vi "Queue_Management_AMC_ALT.vi"(6 "queue error in":errorcluster, 8 "system error in":errorcluster, 9 "Case":string, 10 "Elementos a cola":string[](array[string]), 11 "message queue in":T1) -> (0 "system error out":errorcluster, 2 "elements in queue":cluster{"Estado":string, "Dato":string}[](array[cluster]), 3 "message queue out":T1, 4 "queue error out":errorcluster)   [LabVIEW 2017]
uses:
  <vilib>/NI/AMC/Message Queue.ctl
  <vilib>/NI/AMC/Message.ctl
  <vilib>/NI/Tools/Keyed Array/KeyedArray.ctl
  <vilib>/NI/AMC/Create Single Message.vi
  <vilib>/NI/AMC/Update Message Routing Info.vi
  <vilib>/NI/AMC/Send Message.vi
  <vilib>/NI/AMC/AMC.lvlib
  <vilib>/NI/Tools/Keyed Array/Tools_KeyedArray.lvlib
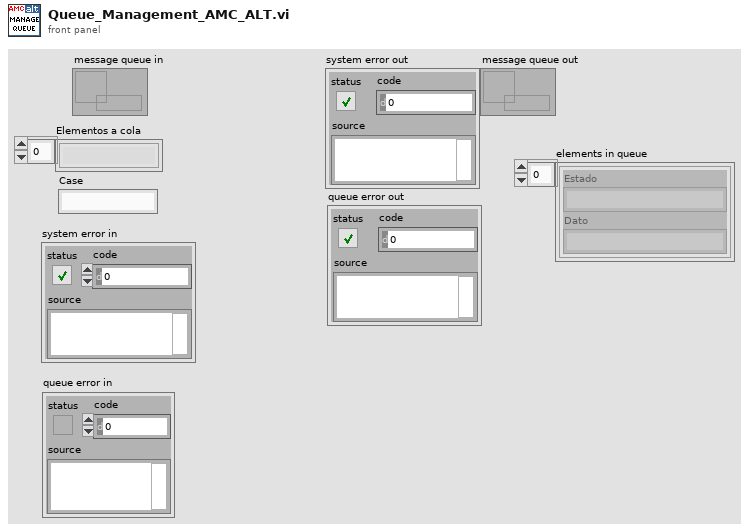
[diagram p1: front panel]
types:
  T1 = typedef "AMC.lvlib/Message Queue.ctl" = refnum<queue>
  T2 = typedef "AMC.lvlib/Message.ctl" = cluster{"name":string, "value":string, "attributes":T3, "receiver host":string, "receiver process":string, "source host":string, "source process":string, "priority message":bool, "acknowledge message":bool}
  T3 = typedef "Tools_KeyedArray.lvlib/KeyedArray.ctl" = cluster{"keys":string[], "values":string[]}
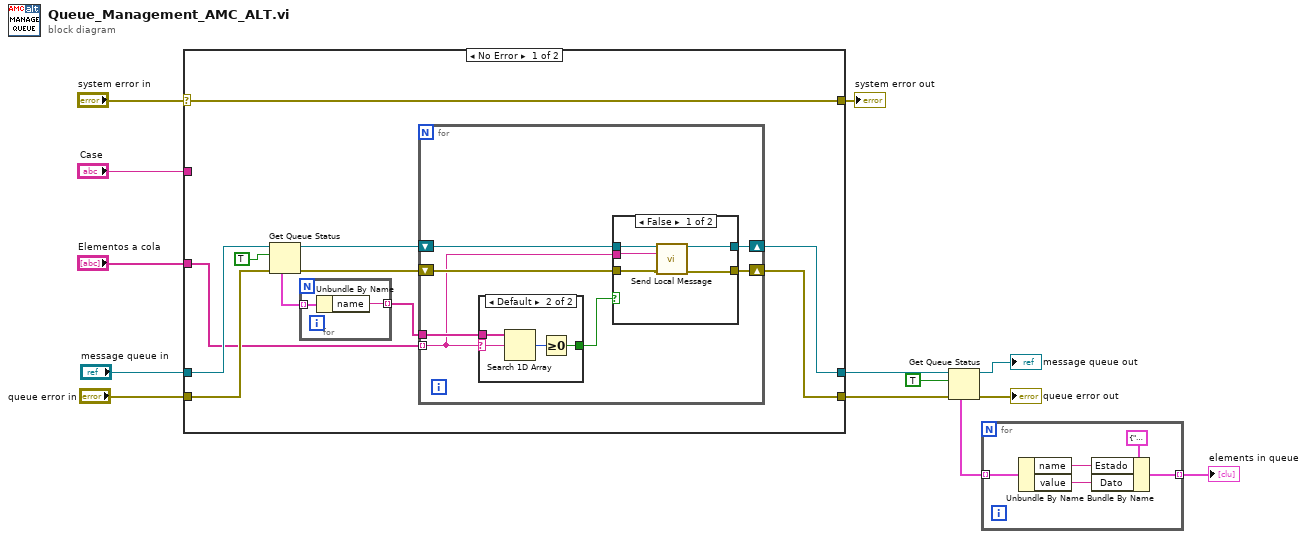
[diagram p0: block diagram]
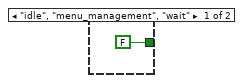
[diagram p2: hidden frame]
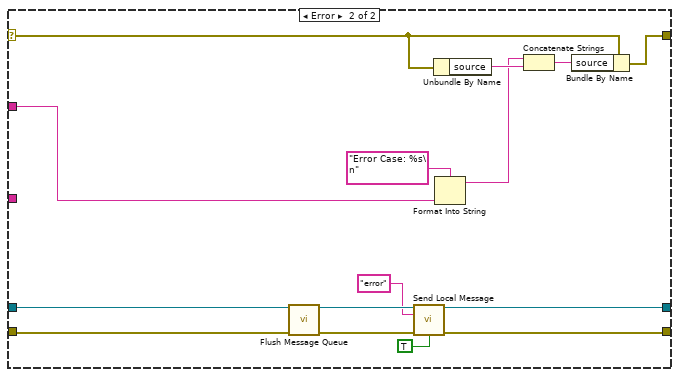
[diagram p4: hidden frame]
diagram:
  n1 = case shown="No Error" "system error in" {
    selector: "system error in" -> [w22 w55]
    tunnel: [w23 w50] -> w4
    tunnel: "Elementos a cola" -> [w16 _]
    tunnel: "message queue in" -> [w18 w52]
    tunnel: [w24 w48] -> w5
    tunnel: "queue error in" -> [w20 w53]
    tunnel: [w22 w56] -> w8
    tunnel: "Case" -> [_ w54]
    frame No Error {
      n2 = Get Queue Status(queue=w18, return elements? (F)=TRUE, error in (no error)=w20) -> (queue out=w17:T1, error out=w19:errorcluster, elements=w15:T2[])  [unwired: 5 out]
      n3 = for {
        tunnel: w15 -> [w26] mode=indexing
        tunnel: [w25] -> w14 mode=indexing
        n4 = Unbundle By Name(w26) -> ("name"=w25:string)
      }
      n5 = for {
        shift-right: [w33] -> w24
        shift-left: w17 -> [w32]
        shift-right: [w30] -> w23
        shift-left: w19 -> [w31]
        tunnel: w14 -> [w28]
        tunnel: w16 -> [w27] mode=indexing
        n6 = case shown="Default" w27 {
          selector: w27 -> [_ w35]
          tunnel: [FALSE w38] -> w29
          tunnel: w28 -> [_ w36]
          frame "idle", "menu_management", "wait" {
          }
          frame Default {
            n7 = Search 1D Array(1D array=w36, element=w35) -> (index of element=w37:i32)  [unwired: 1 in]
            n8 = Greater Or Equal To 0?(x=w37) -> (x >= 0?=w38:bool)
          }
        }
        n9 = case shown="False" w29 {
          tunnel: [w40 w45] -> w33
          tunnel: w32 -> [w43 w45]
          tunnel: w31 -> [w42 w44]
          tunnel: [w39 w44] -> w30
          tunnel: w27 -> [w41 _]
          frame False {
            n10 = call <vilib>:"Send Local Message.vi"("message queue in"=w43, "message name"=w41, "error in"=w42) -> ("message queue out"=w40:T1, "error out"=w39:errorcluster)  [unwired: 10 in, 1 out]
          }
          frame True {
          }
        }
      }
    }
    frame Error {
      n11 = call <vilib>:"Flush Message Queue.vi"("message queue in"=w52, "error in"=w53) -> ("message queue out"=w49:T1, "error out"=w51:errorcluster)  [unwired: 11 in, 1 out]
      n12 = call <vilib>:"Send Local Message.vi"("message queue in"=w49, "message name"="error" ("element"), "error in"=w51, "priority message (F)"=TRUE) -> ("message queue out"=w48:T1, "error out"=w50:errorcluster)  [unwired: 9 in, 1 out]
      n13 = Unbundle By Name(w55) -> ("source"=w59:string)
      n14 = Format Into String(format string="Error Case: %s\n", w54) -> (resulting string=w58:string)  [unwired: 2 in, 1 out]
      n15 = Concatenate Strings(w58, w59) -> (w60:string)
      n16 = Bundle By Name(cluster=w55, "source"=w60) -> (w56:errorcluster)
    }
  }
  "system error out" <- w8
  n17 = Get Queue Status(queue=w5, return elements? (F)=TRUE, error in (no error)=w4) -> (queue out=→"message queue out":T1, error out=→"queue error out":errorcluster, elements=w2:T2[])  [unwired: 5 out]
  n18 = for {
    tunnel: w2 -> [w65] mode=indexing
    tunnel: [w61] -> w1 mode=indexing
    n19 = Unbundle By Name(w65) -> ("name"=w63:string, "value"=w62:string)
    n20 = Bundle By Name(cluster=cluster{"Estado":string, "Dato":string} {"Estado"="", "Dato"=""} ("Cluster"), "Estado"=w63, "Dato"=w62) -> (w61:cluster{"Estado":string, "Dato":string})
  }
  "elements in queue" <- w1
